vi "CreateEvent.vi"(10 "EQ_Name":string, 11 "EventRef":refnum<data-value>) -> (3 "Data Value Reference out":refnum<data-value>)   [LabVIEW 2014]
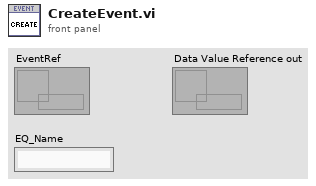
[diagram p1: front panel]
types:
  T1 = cluster{"CmdMsg":cluster{"msg":string, "data":variant}, "EQ_Name":string, "user event out":refnum<user-event>}
  T2 = cluster{"CmdMsg":cluster{"msg":string, "data":variant}, "EQ_Name":string, "user event out":refnum<user-event>}[]
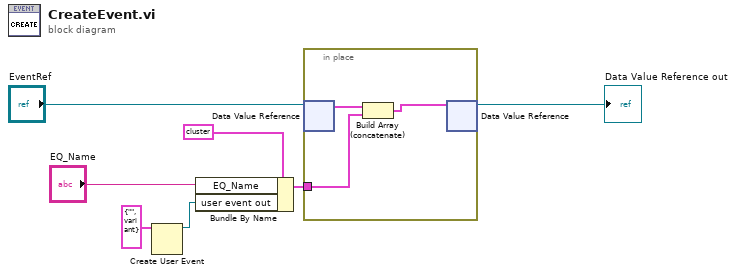
[diagram p0: block diagram]
diagram:
  n1 = Create User Event(user event datatype=cluster{"msg":string, "data":variant} {"msg"="", "data"=variant} ("CmdMsg")) -> (user event=w6:refnum<user-event>)  [unwired: 1 in, 1 out]
  n2 = Bundle By Name(cluster=T1 {"CmdMsg"={"msg"="", "data"=variant}, "EQ_Name"="", "user event out"=refnum} ("output cluster"), "EQ_Name"="EQ_Name", "user event out"=w6) -> (w2:T1)
  n3 = in-place {
    in-place-border: w2 -> [w9]
    n4 = in-place-dvr #1("EventRef") -> (w10:T2)  [unwired: 1 out]
    n5 = Build Array (concatenate)(w10, w9) -> (w8:T2)
    n6 = in-place-dvr #1(w8) -> (→"Data Value Reference out":refnum<data-value>)  [unwired: 1 out]
  }
